vi "Pack Auto-Launch Models Msg.vi"(6 "Confirm Shutdown? (T)":bool=TRUE, 9 "Auto-stop? (T)":bool=TRUE, 10 "Models":refnum<class "IModel.lvclass">[](array[class])) -> (3 "Launch Nested Models Msg":refnum<class "Auto-Launch Models Msg.lvclass">)   [LabVIEW 2020, in "MVA Framework.lvlib" / "IModel.lvlib" / "Auto-Launch Models Msg.lvclass"]
doc: "打包自动启动模型消息"
uses:
  Auto-Launch Models Msg.lvclass
  IModel/IModel.lvclass
  C:/Program Files/National Instruments/LabVIEW 2020/vi.lib/ActorFramework/Actor/Actor.lvclass
  Auto-Launch Models Msg.lvclass/Auto-Launch Models Msg.ctl
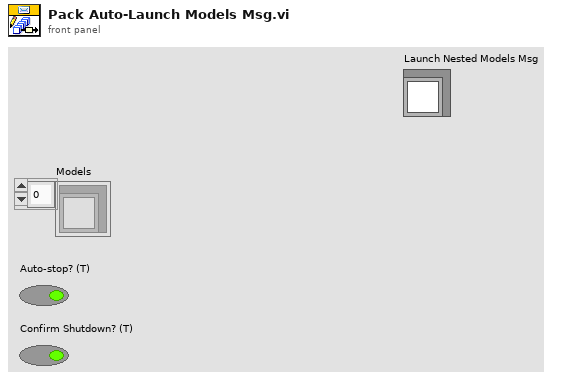
[diagram p1: front panel]
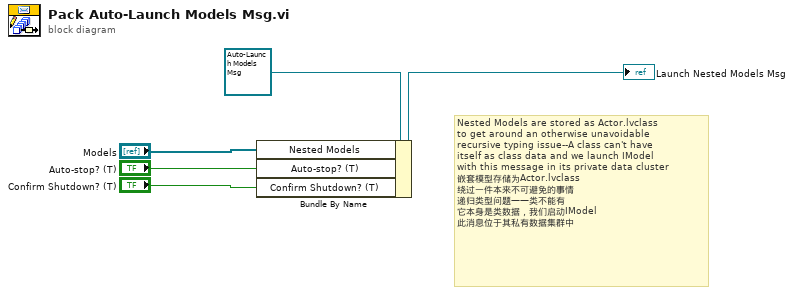
[diagram p0: block diagram]
diagram:
  # "Nested Models are stored as Actor.lvclass\nto get around an otherwise unavoidable\nrecursive typing issue--A class can't have\nitself as class data and we launch IModel\nwith this message in its private data cluster\n嵌套模型存储为Actor.lvclass\n绕过一件本来不可避免的事情\n递归类型问题——类不能有\n它本身是类数据，我们启动IModel\n此消息位于其私有数据集群中"
  n1 = Bundle By Name(cluster=refnum<class "Auto-Launch Models Msg.lvclass"> refnum ("Launch Nested Models Msg"), "Nested Models"="Models", "Auto-stop? (T)"="Auto-stop? (T)", "Confirm Shutdown? (T)"="Confirm Shutdown? (T)") -> (→"Launch Nested Models Msg":refnum<class "Auto-Launch Models Msg.lvclass">)
